vi "Test Customer Pick Up Last Order Item Stops if in App Context.vi"(8 "error in (no error)":errorcluster, 11 "Customer Test in":refnum<class "Customer Test.lvclass">) -> (0 "error out":errorcluster, 3 "Customer Test out":refnum<class "Customer Test.lvclass">)   [LabVIEW 2020, in "Customer Test.lvclass"]
uses:
  Customer Test.lvclass
  C:/Program Files (x86)/National Instruments/LabVIEW 2020/vi.lib/Asteme/LUnit/Test Case.lvclass
  Customer/Customer.lvclass
  C:/Program Files (x86)/National Instruments/LabVIEW 2020/vi.lib/Asteme/Triarc Framework/Process/Process.lvclass
  Support/Beverages/Beverage/Beverage.lvclass
  Support/Beverages/TypeDefs/Drink Type.ctl
  Support/Beverages/TypeDefs/Options.ctl
  <vilib>/Asteme/Triarc Framework/Process/Public/Lifecycle/Lifecycle State.ctl
  <vilib>/Asteme/Triarc Framework/Application/Application.lvclass
  Stub Job Processor/Stub Job Handler.lvclass
  C:/Users/anton/Documents/GitHub/Triarc-Examples/Coffee Shop/Process Job/Job Handler.lvclass
  <vilib>/Asteme/LUnit/Test Case.lvclass/Test Case.ctl
  <vilib>/Asteme/LUnit/LUnit Assertion Result.lvclass/LUnit Assertion Result.ctl
  <vilib>/Asteme/Triarc Framework/Process/Process.lvclass/Process.ctl
  <vilib>/Asteme/Triarc Framework/Application/Application.lvclass/Application.ctl
  <vilib>/Asteme/Triarc Framework/Application/Private/Add Process to Map.vi
  <vilib>/Asteme/Triarc Framework/Application/Private/Start Idle Processes if Running.vi
  <vilib>/Asteme/Triarc Framework/Process/Protected/Messaging/Enqueue Message.vi
  <vilib>/Asteme/Triarc Framework/Process/Public/Lifecycle/Get Lifecycle State.vi
  <vilib>/Asteme/Triarc Framework/Process/Protected/SubVIs/Set Context.vi
  <vilib>/Asteme/LUnit/Palette/Pass If.vi
  <vilib>/Asteme/LUnit/Set Assertion Type.vi
  <vilib>/Asteme/Triarc Framework/Process/Private/SubVIs/Wait for finish.vi
  <vilib>/Asteme/Triarc Framework/Process/Private/SubVIs/Set Lifecycle State.vi
  <vilib>/Utility/error.llb/Clear Errors.vi
  <vilib>/AdvancedString/1D String Array to Delimited String.vi
  <vilib>/Asteme/Triarc Framework/Process/Public/Lifecycle/Leave Process Loop.vi
  <vilib>/Asteme/LUnit/Palette/Fail.vi
  <vilib>/Asteme/LUnit/Palette/Pass.vi
  <vilib>/Asteme/LUnit/LUnit Write Assertion Type.vi
  <vilib>/Asteme/LUnit/Add test result.vi
  <vilib>/Asteme/LUnit/LUnit Write Passed.vi
  <vilib>/Asteme/LUnit/LUnit Get Test Case.vi
  <vilib>/Asteme/LUnit/Assertion Result/LUnit Get Test Name.vi
  <vilib>/Asteme/LUnit/LUnit Write Message.vi
  <vilib>/Asteme/LUnit/LUnit Write Description.vi
  <vilib>/Asteme/LUnit/Read Test Case Name.vi
  <vilib>/Utility/error.llb/Error Cluster From Error Code.vi
  <vilib>/Asteme/Triarc Framework/Application/Private/Update Context for Owned Processes.vi
  <vilib>/Asteme/LUnit/LUnit Assertion Result.lvclass
  <vilib>/Asteme/Triarc Framework/Process/Process.lvclass
  <vilib>/Asteme/LUnit/Test Case.lvclass
  C:/Program Files (x86)/National Instruments/LabVIEW 2020/vi.lib/Asteme/Triarc Framework/Base/Base.lvclass
  C:/Program Files (x86)/National Instruments/LabVIEW 2020/vi.lib/Asteme/Triarc Framework/Error Handler Interface/Error Handler Interface.lvclass
  C:/Program Files (x86)/National Instruments/LabVIEW 2020/vi.lib/Asteme/Triarc Framework/Logging/Logging.lvclass
  C:/Program Files (x86)/National Instruments/LabVIEW 2020/vi.lib/Asteme/Triarc Framework/Application/Application.lvclass
  C:/Users/anton/Documents/GitHub/Triarc-Examples/Coffee Shop/Person/Person.lvclass
  C:/Program Files (x86)/National Instruments/LabVIEW 2020/vi.lib/Asteme/Triarc Framework/View/View.lvclass
  C:/Users/anton/Documents/GitHub/Triarc-Examples/Coffee Shop/Customer/Customer.lvclass
  C:/Program Files (x86)/National Instruments/LabVIEW 2020/vi.lib/Asteme/Triarc Framework/Asynchronous Action/Async Action.lvclass
  C:/Users/anton/Documents/GitHub/Triarc-Examples/Coffee Shop/Stub Job Processor/Stub Job Handler.lvclass
  C:/Users/anton/Documents/GitHub/Triarc-Examples/Coffee Shop/Person Test/Person Test.lvclass
  C:/Program Files (x86)/National Instruments/LabVIEW 2020/vi.lib/Asteme/Triarc Framework Test Suite/View Test/View Test.lvclass
  C:/Program Files (x86)/National Instruments/LabVIEW 2020/vi.lib/Asteme/Triarc Framework Test Suite/Process Test/Process Test.lvclass
  C:/Program Files (x86)/National Instruments/LabVIEW 2020/vi.lib/Asteme/Triarc Framework Test Suite/Base Class Test/Base Test.lvclass
  C:/Users/anton/Documents/GitHub/Triarc-Examples/Coffee Shop/Customer Test/Customer Test.lvclass
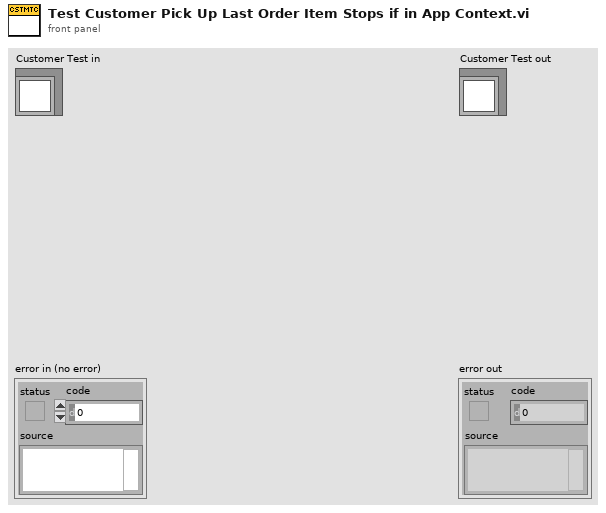
[diagram p1: front panel]
types:
  T1 = typedef "TF.lvlib/Process.lvclass/Lifecycle State.ctl" = enum16{"Uninitialized", "Initialized", "Started", "Running", "Stopped", "Finished"}
  T2 = typedef "Beverage.lvclass/Drink Type.ctl" = enum16{"Dark Roast", "Decaf", "Espresso", "House Blend"}
  T3 = typedef "Beverage.lvclass/Options.ctl" = enum16{"<None>", "Milk", "Mocha", "Soy", "Whip"}
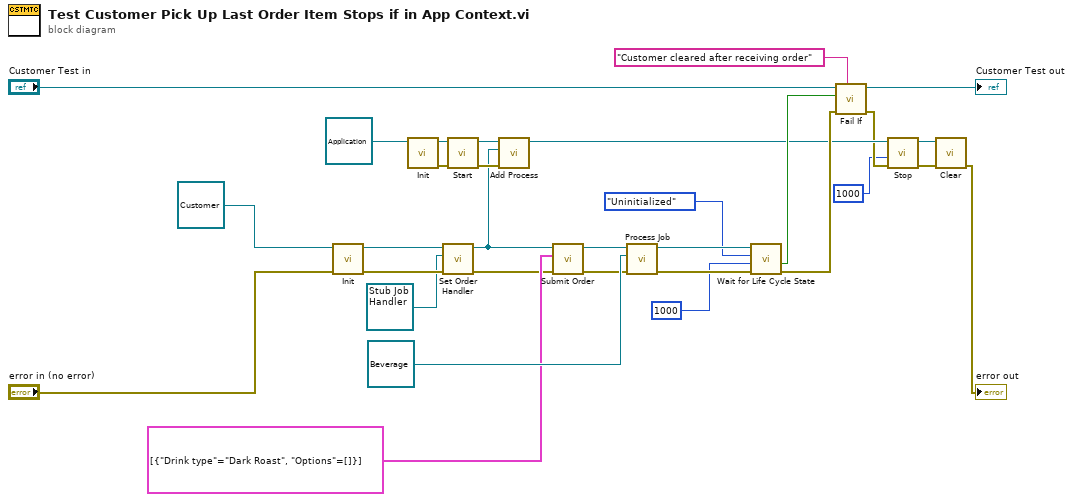
[diagram p0: block diagram]
diagram:
  n1 = call-dynamic "Init.vi"("error in (no error)"="error in (no error)", "View In"=refnum<class "Customer.lvclass"> refnum ("Customer.lvclass")) -> ("error out"=w30:errorcluster, "View Out"=w3:refnum<class "Customer.lvclass">)  [unwired: 8 in]
  n2 = call-dynamic "Init.vi"("Process In"=refnum<class "Application.lvclass"> refnum ("TF.lvlib:Application.lvclass")) -> ("error out"=w14:errorcluster, "Process Out"=w15:refnum<class "Application.lvclass">)  [unwired: 9 in]
  n3 = call "Set Order Handler.vi"("error in (no error)"=w30, "Order Handler"=refnum<class "Stub Job Handler.lvclass"> refnum ("Stub Job Handler.lvclass"), "Customer In"=w3) -> ("error out"=w4:errorcluster, "Customer Out"=w2:refnum<class "Customer.lvclass">)  [unwired: 7 in]
  n4 = call <vilib>:"Start.vi"("error in (no error)"=w14, "Process In"=w15) -> ("error out"=w11:errorcluster, "Process Out"=w12:refnum<class "Application.lvclass">)  [unwired: 8 in]
  n5 = call <vilib>:"Add Process.vi"("error in (no error)"=w11, "Process"=w2, "Rig In"=w12) -> ("Rig Out"=w10:refnum<class "Application.lvclass">)  [unwired: 7 in, 1 out]
  n6 = call "Submit Order.vi"("error in (no error)"=w4, "Order Content"=cluster{"Drink type":T2, "Options":T3[]}[] [{"Drink type"=enum."Dark Roast", "Options"=[]}], "Customer In"=w2) -> ("error out"=w21:errorcluster, "Customer Out"=w20:refnum<class "Customer.lvclass">)  [unwired: 7 in]
  n7 = call-dynamic "Process Job.vi"("error in (no error)"=w21, "Task"=refnum<class "Beverage.lvclass"> refnum ("Beverage.lvclass"), "Work Dispatcher In"=w20) -> ("error out"=w28:errorcluster, "Work Dispatcher Out"=w22:refnum<class "Customer.lvclass">)  [unwired: 7 in]
  n8 = call <vilib>:"Wait for Life Cycle State.vi"("error in (no error)"=w28, "timeout in ms (-1)"=1000, "Lifecycle State"=Lifecycle_State."Uninitialized", "Process In"=w22) -> ("error out"=w23:errorcluster, "timed out?"=w16:bool)  [unwired: 5 in, 1 out]
  n9 = call <vilib>:"Fail If.vi"("Description"="Customer cleared after receiving order", "error in (no error)"=w23, "Fail?"=w16, "Test Case In"="Customer Test in") -> ("error out"=w7:errorcluster, "Test Case Out"=→"Customer Test out":refnum<class "Customer Test.lvclass">)  [unwired: 6 in]
  n10 = call <vilib>:"Stop.vi"("error in (no error)"=w7, "timeout in ms (-1)"=1000, "Process In"=w10) -> ("error out"=w8:errorcluster, "Process Out"=w9:refnum<class "Application.lvclass">)  [unwired: 6 in, 1 out]
  n11 = call-dynamic "Clear.vi"("error in (no error)"=w8, "Application In"=w9) -> ("error out"=→"error out":errorcluster)  [unwired: 9 in]
